vi "FTW-Actor-CheckShutdown.vi"(0 "FTW Actor in":refnum<class "FTW-Actor.lvclass">, 11 "error in":errorcluster) -> (4 "FTW Actor":refnum<class "FTW-Actor.lvclass">, 6 "Shutdown?":bool, 15 "error out":errorcluster)   [LabVIEW 2014, in "FTW-Actor.lvclass"]
uses:
  FTW-Actor.lvclass
  Sequencer/FTW-Sequencer.lvclass
panel:
  # "Inputs"
  # "Outputs"
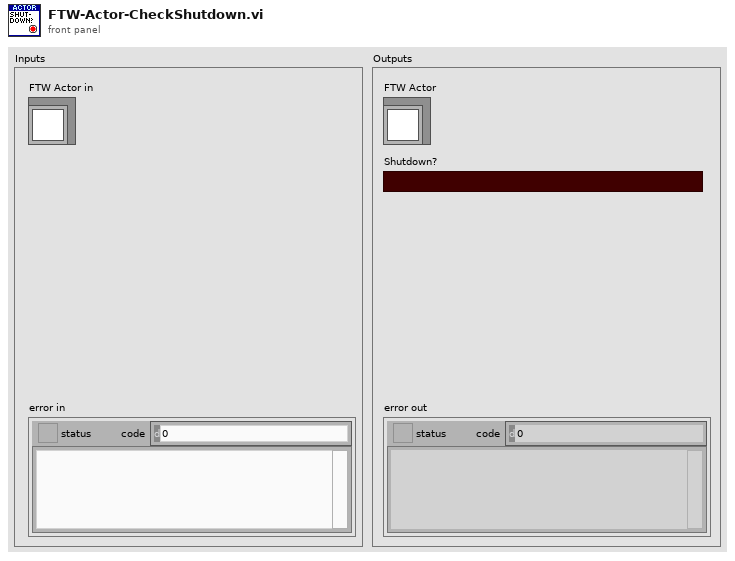
[diagram p1: front panel]
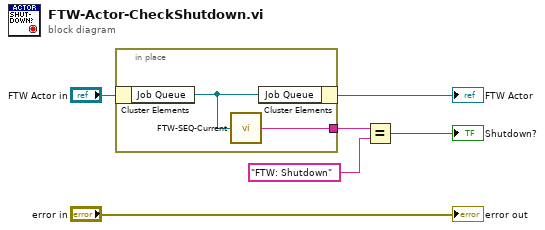
[diagram p0: block diagram]
diagram:
  n1 = in-place {
    in-place-border: [w7] -> w3
    n2 = in-place-cluster #1("FTW Actor in") -> ("Job Queue"=w8:refnum<class "FTW-Sequencer.lvclass">)
    n3 = call "FTW-SEQ-Current.vi"("Sequencer"=w8) -> ("Current Job"=w7:string)
    n4 = in-place-cluster #1("Job Queue"=w8) -> (→"FTW Actor":refnum<class "FTW-Actor.lvclass">)
  }
  n5 = Equal?(x=w3, y="FTW: Shutdown") -> (x = y?=→"Shutdown?":bool)
  "error out" <- "error in"
